vi "ADSR_Envelope_Generation_subVI.vi"(8 "ADSR Envelope Cluster in":T1, 11 "Number of Samples in":dbl) -> (0 "Envelope XY Graph out":cluster{dbl[], dbl[]}, 3 "Envelope Array out":dbl[](array[numeric]))   [LabVIEW 2019]
doc: "This SubVI takes the number of samples, and ADSR Envelope Cluster info. From this info, subVI creates an array of amplitude (MIN = 0, MAX = 1) for every sample acording to the ADSR variables.\nSubVI also creates a XY graph of created envelope.\n\nIN: ADSR Envelope Cluster; Number of samples;\nOUT: Envelope Array, Envelope XY Graph;"
panel:
  out "Debug XY graph":cluster{dbl[], dbl[]}(graph)
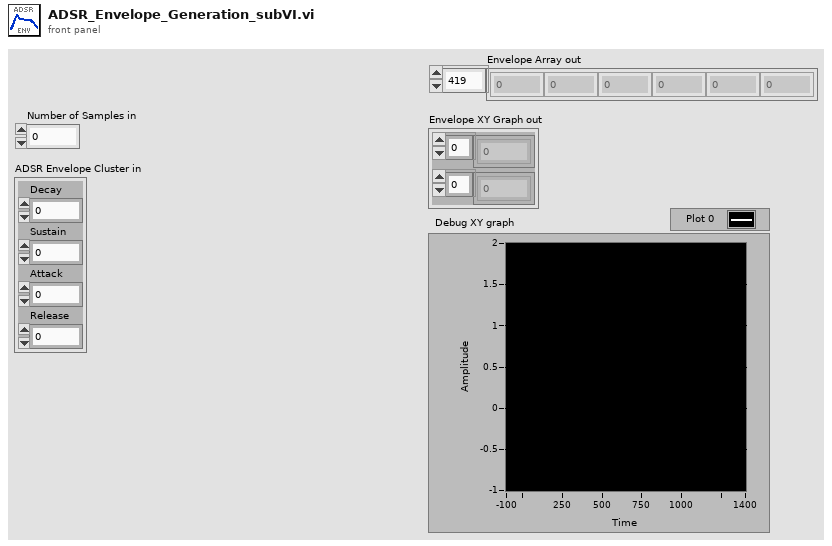
[diagram p1: front panel]
types:
  T1 = cluster{"Decay":i32, "Sustain":i32, "Attack":i32, "Release":i32}
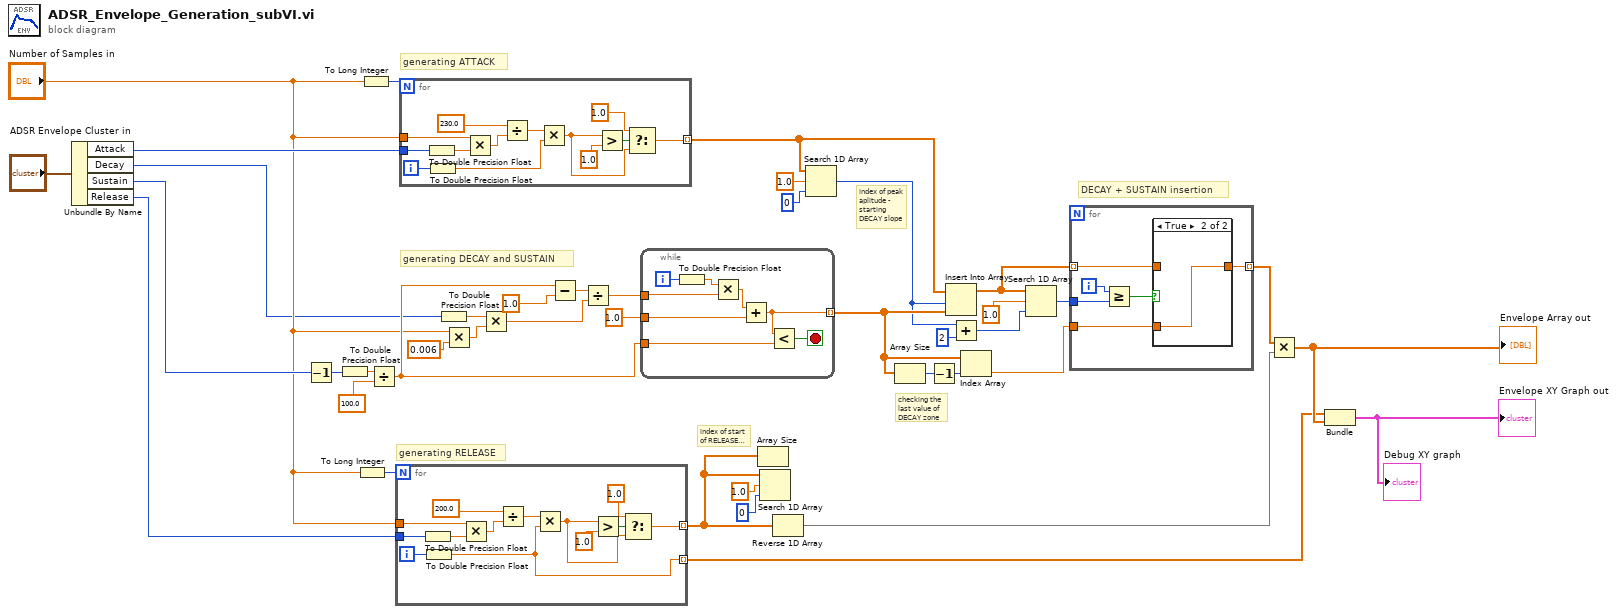
[diagram p0: block diagram]
diagram:
  # "DECAY + SUSTAIN insertion"
  # "generating DECAY and SUSTAIN"
  # "checking the last value of DECAY zone"
  # "index of start of RELEASE zone"
  # "index of peak aplitude - starting DECAY slope"
  # "generating ATTACK"
  # "generating RELEASE"
  n1 = Unbundle By Name("ADSR Envelope Cluster in") -> ("Attack"=w9:i32, "Decay"=w1:i32, "Sustain"=w8:i32, "Release"=w7:i32)
  n2 = Decrement(x=w8) -> (x-1=w11:i32)
  n3 = To Double Precision Float(number=w11) -> (double precision float=w30:dbl)
  n4 = To Long Integer(number="Number of Samples in") -> (32bit integer=w39:i32)
  n5 = To Long Integer(number="Number of Samples in") -> (32bit integer=w38:i32)
  n6 = Divide(x=w30, y=100.0) -> (x/y=w25:dbl)
  n7 = for {
    N: w39 -> [_]
    tunnel: [w48] -> w32 mode=indexing
    tunnel: "Number of Samples in" -> [w47]
    tunnel: [w45] -> w24 mode=indexing
    tunnel: w7 -> [w44]
    i -> [w54]
    n8 = To Double Precision Float(number=w44) -> (double precision float=w46:dbl)
    n9 = To Double Precision Float(number=w54) -> (double precision float=w45:dbl)
    n10 = Multiply(x=w47, y=w46) -> (x*y=w51:dbl)
    n11 = Divide(x=200.0, y=w51) -> (x/y=w50:dbl)
    n12 = Multiply(x=w50, y=w45) -> (x*y=w49:dbl)
    n13 = Greater?(x=w49, y=1.0) -> (0:w53:bool)
    n14 = Select(t=1.0, s=w53, f=w49) -> (s? t:f=w48:dbl)
  }
  n15 = for {
    N: w38 -> [_]
    tunnel: [w58] -> w21 mode=indexing
    tunnel: "Number of Samples in" -> [w57]
    tunnel: w9 -> [w55]
    i -> [w67]
    n16 = To Double Precision Float(number=w55) -> (double precision float=w56:dbl)
    n17 = To Double Precision Float(number=w67) -> (double precision float=w60:dbl)
    n18 = Multiply(x=w57, y=w56) -> (x*y=w62:dbl)
    n19 = Divide(x=230.0, y=w62) -> (x/y=w61:dbl)
    n20 = Multiply(x=w61, y=w60) -> (x*y=w59:dbl)
    n21 = Greater?(x=w59, y=1.0) -> (0:w66:bool)
    n22 = Select(t=1.0, s=w66, f=w59) -> (s? t:f=w58:dbl)
  }
  n23 = To Double Precision Float(number=w1) -> (double precision float=w2:dbl)
  n24 = Multiply(x="Number of Samples in", y=0.006) -> (x*y=w4:dbl)
  n25 = Multiply(x=w2, y=w4) -> (x*y=w3:dbl)
  n26 = Subtract(x=w25, y=1.0 ("x")) -> (x-y=w29:dbl)
  n27 = Divide(x=w29, y=w3) -> (x/y=w28:dbl)
  n28 = while {
    tunnel: [w68] -> w20 mode=indexing
    tunnel: 1.0 -> [w72]
    tunnel: w28 -> [w73]
    tunnel: w25 -> [w69]
    i -> [w71]
    stop <- w70 stop-if-true
    n29 = To Double Precision Float(number=w71) -> (double precision float=w75:dbl)
    n30 = Multiply(x=w75, y=w73) -> (x*y=w74:dbl)
    n31 = Add(x=w74, y=w72) -> (x+y=w68:dbl)
    n32 = Less?(x=w68, y=w69) -> (x < y?=w70:bool)
  }
  n33 = Array Size(array=w32) -> ()  [unwired: 1 out]
  n34 = Search 1D Array(1D array=w32, element=1.0, start index (0)=0) -> ()  [unwired: 1 out]
  n35 = Reverse 1D Array(array=w32) -> (reversed array=w40:dbl[])
  n36 = Search 1D Array(1D array=w21, element=1.0, start index (0)=0) -> (index of element=w18:i32)
  n37 = Array Size(array=w20) -> (size(s)=w23:i32)
  n38 = Decrement(x=w23) -> (x-1=w22:i32)
  n39 = Insert Into Array(array=w21, index=w18, new element=w20) -> (w14:dbl[])
  n40 = Add(x=w18, y=2) -> (x+y=w16:i32)
  n41 = Index Array(array=w20, index=w22) -> (element=w12:dbl)
  n42 = Search 1D Array(1D array=w14, element=1.0, start index (0)=w16) -> (index of element=w15:i32)
  n43 = for {
    tunnel: w15 -> [w80]
    tunnel: w14 -> [w79] mode=indexing
    tunnel: [w78] -> w13 mode=indexing
    tunnel: w12 -> [w77]
    i -> [w76]
    n44 = Greater Or Equal?(x=w76, y=w80) -> (x >= y?=w81:bool)
    n45 = case shown="True" w81 {
      tunnel: w79 -> [w82 _]
      tunnel: [w82 w83] -> w78
      tunnel: w77 -> [_ w83]
      frame False {
      }
      frame True {
      }
    }
  }
  n46 = Multiply(x=w13, y=w40) -> (x*y=w41:dbl[])
  "Envelope Array out" <- w41
  n47 = Bundle(w24, w41) -> (→"Envelope XY Graph out" →"Debug XY graph":cluster{dbl[], dbl[]})  [unwired: 1 in]
